vi "MB_TCP_NS300.vi"(5 "Status Reference":T1, 6 "N":i32, 7 "Data Reference":T2, 9 "timeouts":T3={"conn_timeout"=1000, "reconn_timeout"=3000, "N attempt max"=3, "t_reset_TTL"=120000, "write_timeout"=10, "read_timeout"=500, "period"=100} {"t_reset_TTL" min=10 max=240000 step=1; "period" min=10 max=100000 step=1; "read_timeout" min=10 max=60000 step=1; "write_timeout" min=1 max=60000 step=1; "N attempt max" min=1 max=5 step=1; "reconn_timeout" min=10 max=240000 step=1; "conn_timeout" min=10 max=240000}, 10 "write enable":bool=TRUE, 11 "stop":bool) -> (0 "error out":errorcluster, 2 "errors":i32, 3 "Z3":u32)   [LabVIEW 2019, in "MB_TCP1.lvlib"]
uses:
  MB_TCP1.lvlib
  Timer Delay/Timers.lvlib
  NI_modbus_upd/NI_modbus_upd.lvlib
  NI_modbus_upd/MB Modbus Command.ctl
  ICPCON Registers/ICPCON Registers.lvlib
  ICPCON Status/ICPCON Status.lvlib
  Timer Delay/unix time 1ms.vi
  NI_modbus_upd/TCP/TCP.lvclass
  ICPCON Registers/Ctl/ICPCON Data.ctl
  ICPCON Status/Ctl/ICPCON Status.ctl
panel:
  out "stopped":bool
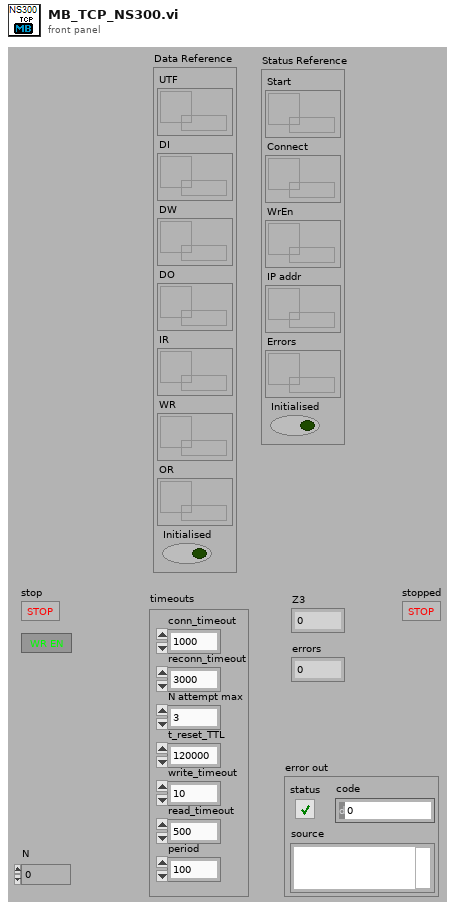
[diagram p1: front panel]
types:
  T1 = typedef "ICPCON Status.lvlib/ICPCON Status.ctl" = cluster{"Start":refnum<data-value>, "Connect":refnum<data-value>, "WrEn":refnum<data-value>, "IP addr":refnum<data-value>, "Errors":refnum<data-value>, "Initialised":bool}
  T2 = typedef "ICPCON Registers.lvlib/ICPCON Data.ctl" = cluster{"UTF":refnum<data-value>, "DI":refnum<data-value>, "DW":refnum<data-value>, "DO":refnum<data-value>, "IR":refnum<data-value>, "WR":refnum<data-value>, "OR":refnum<data-value>, "Initialised":bool}
  T3 = cluster{"conn_timeout":i32, "reconn_timeout":i32, "N attempt max":i32, "t_reset_TTL":i32, "write_timeout":i32, "read_timeout":i32, "period":i32}
  T4 = typedef "NI_modbus_upd.lvlib/MB Modbus Command.ctl" = cluster{"Function Code":u8, "Starting Address":u16, "Quantity":u16, "Data":u16[], "Discrete":bool[]}
  T5 = cluster{"Transaction ID":u16, "Protocol ID":u16, "Length":u16, "Unit ID":u8}
  T6 = cluster{"Remote IP Address":string, "Remote Port":u16}
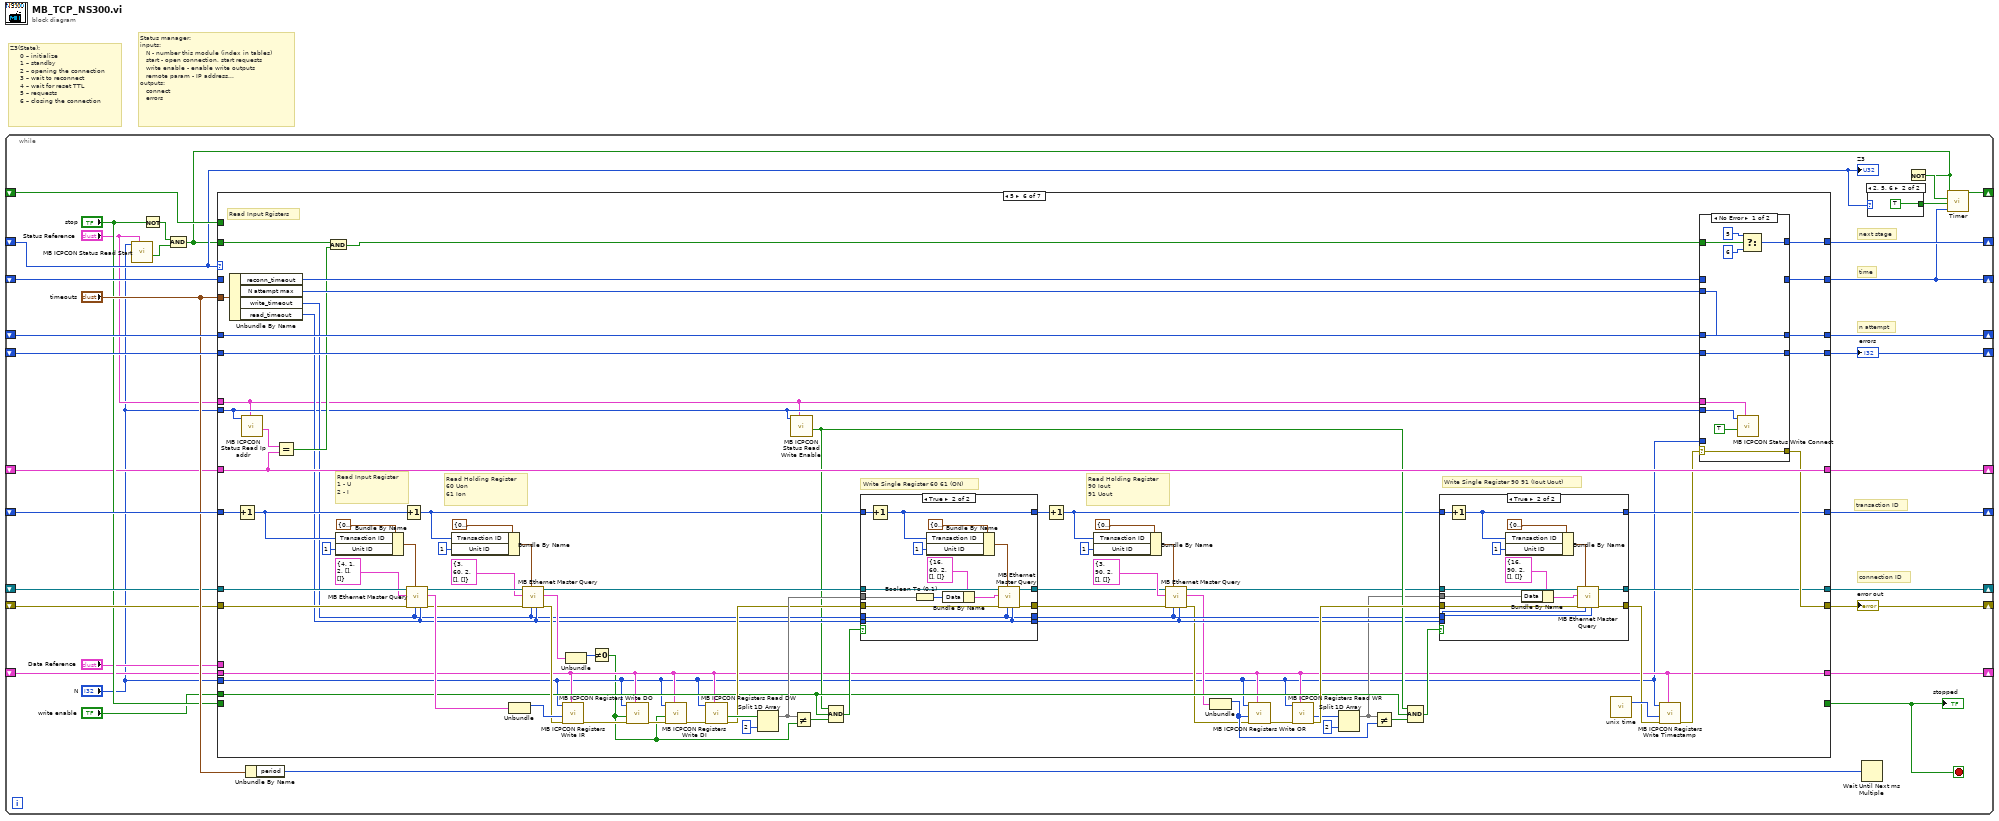
[diagram p0: block diagram]
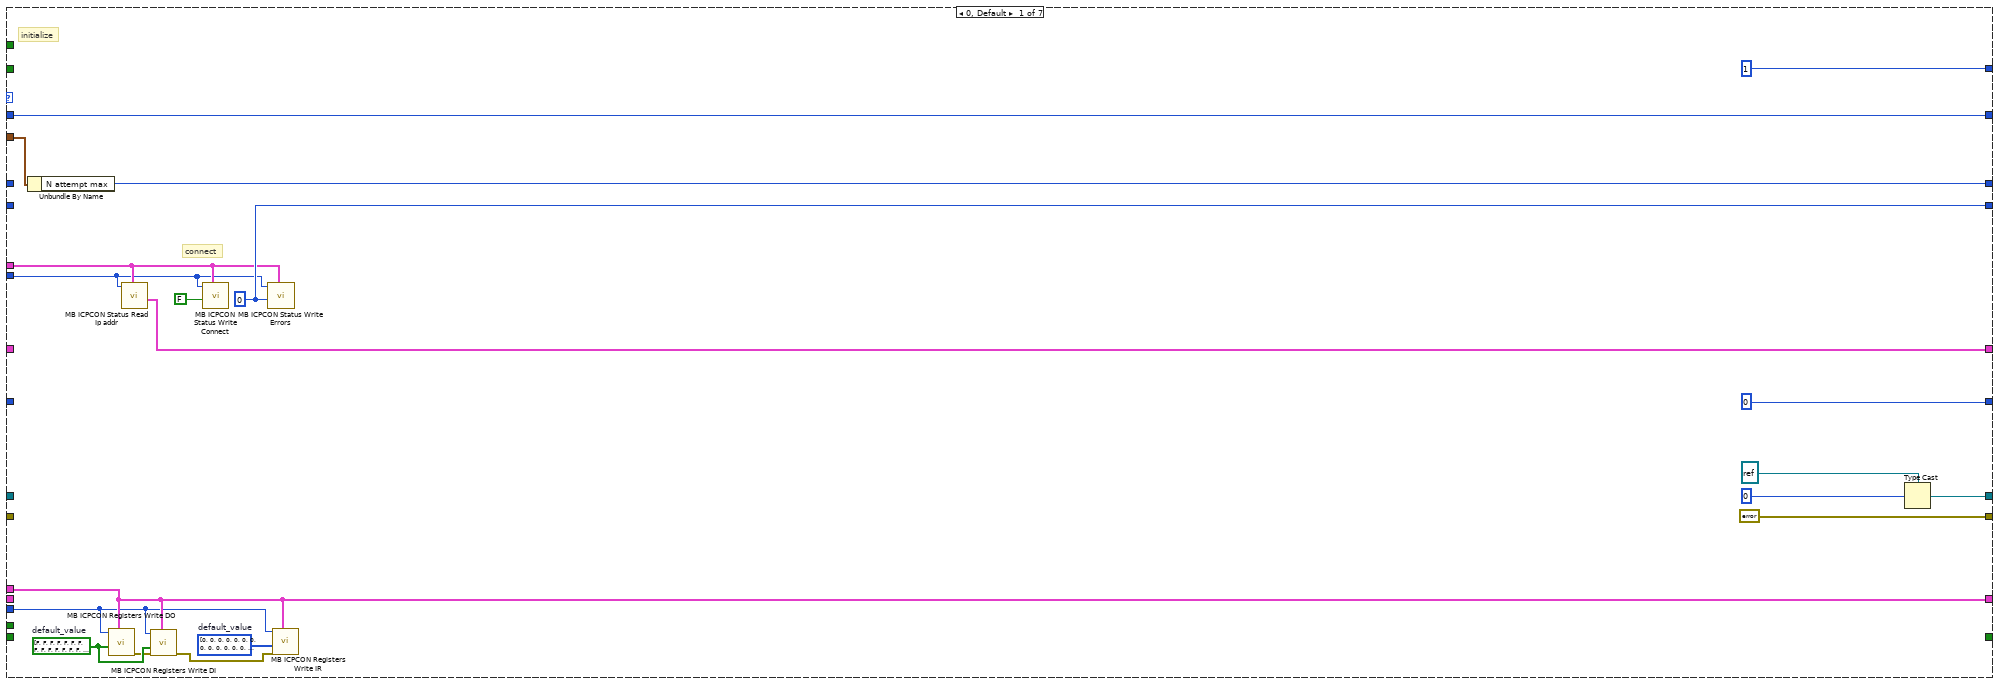
[diagram p2: hidden frame]
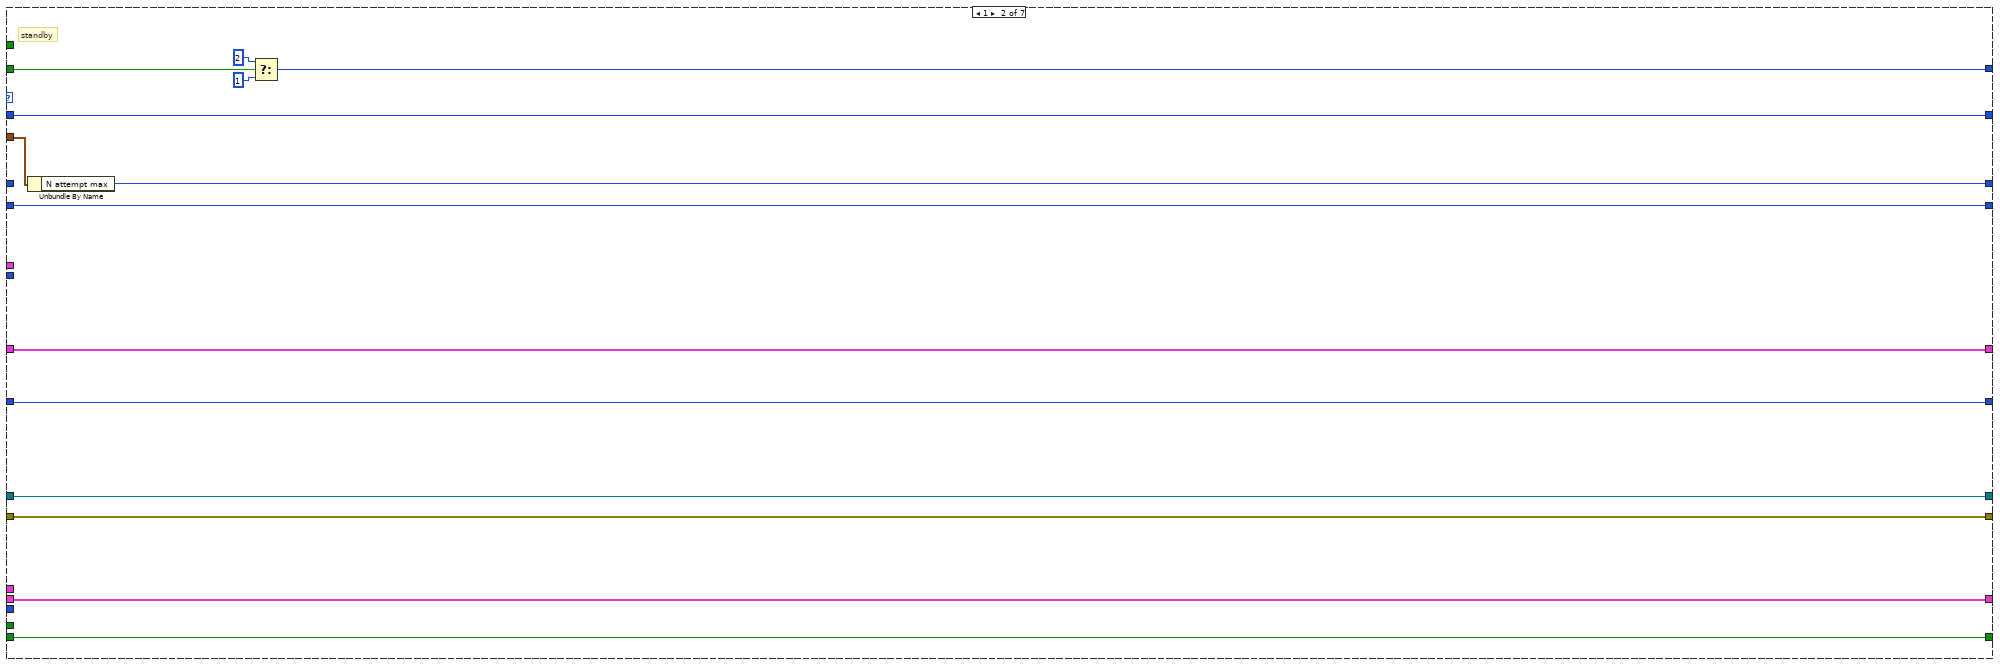
[diagram p3: hidden frame]
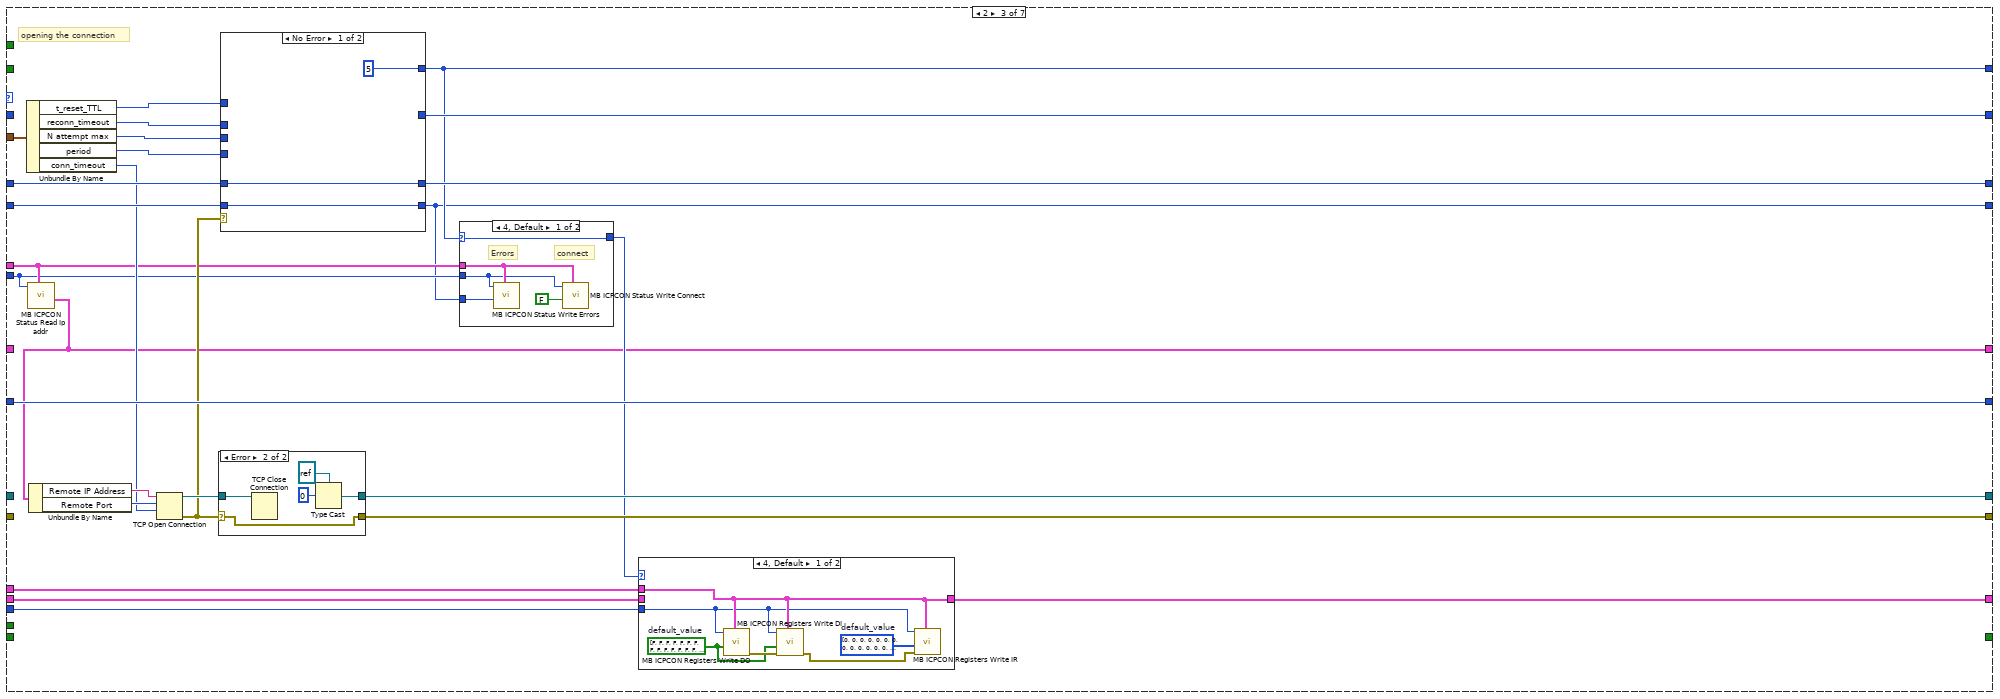
[diagram p4: hidden frame]
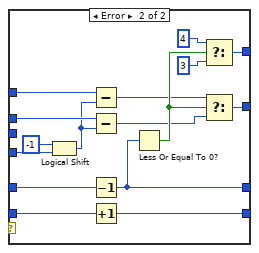
[diagram p8: hidden frame]
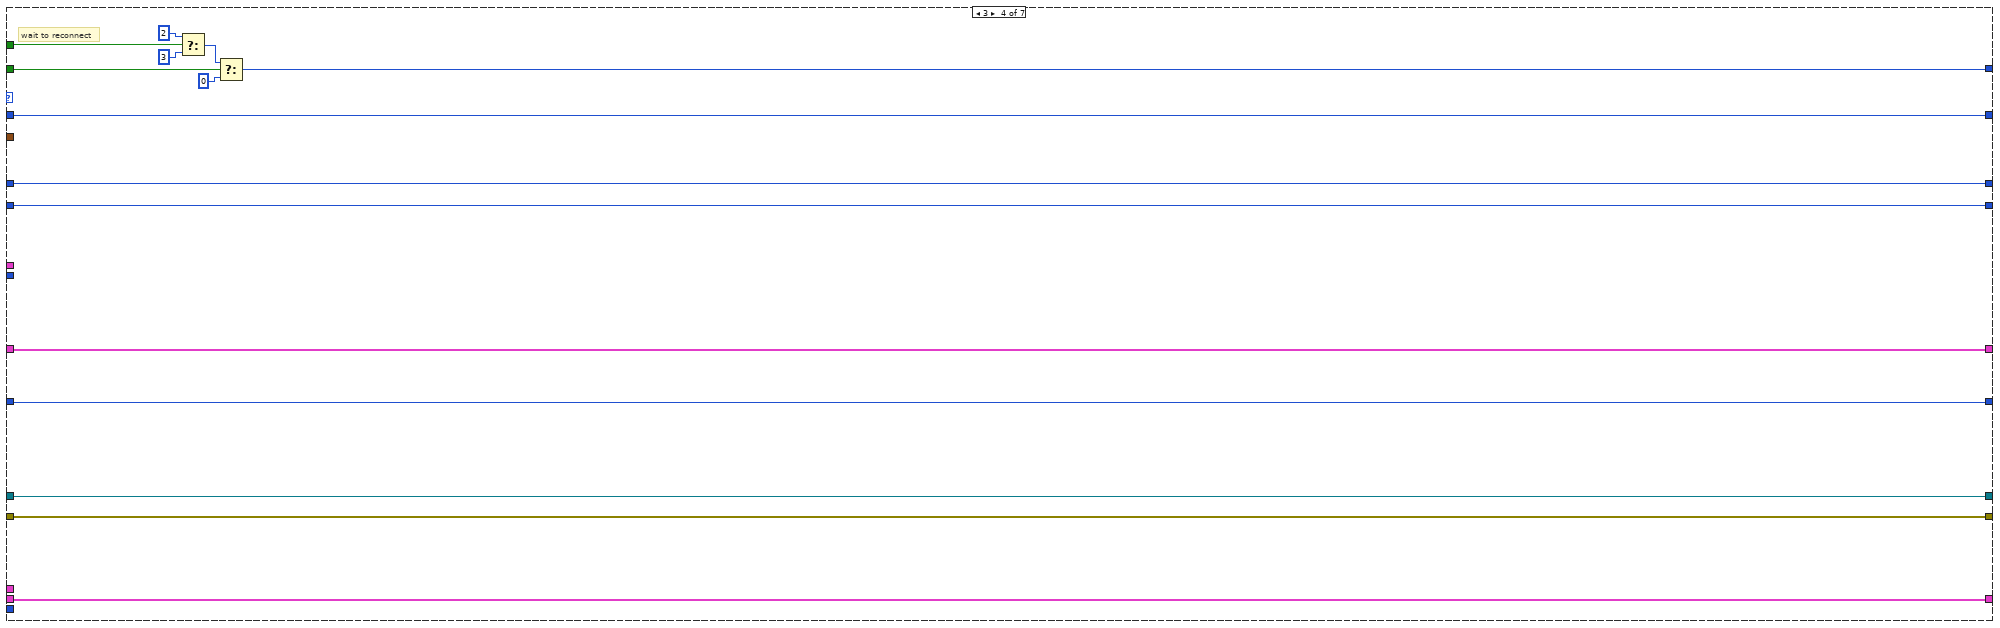
[diagram p9: hidden frame]
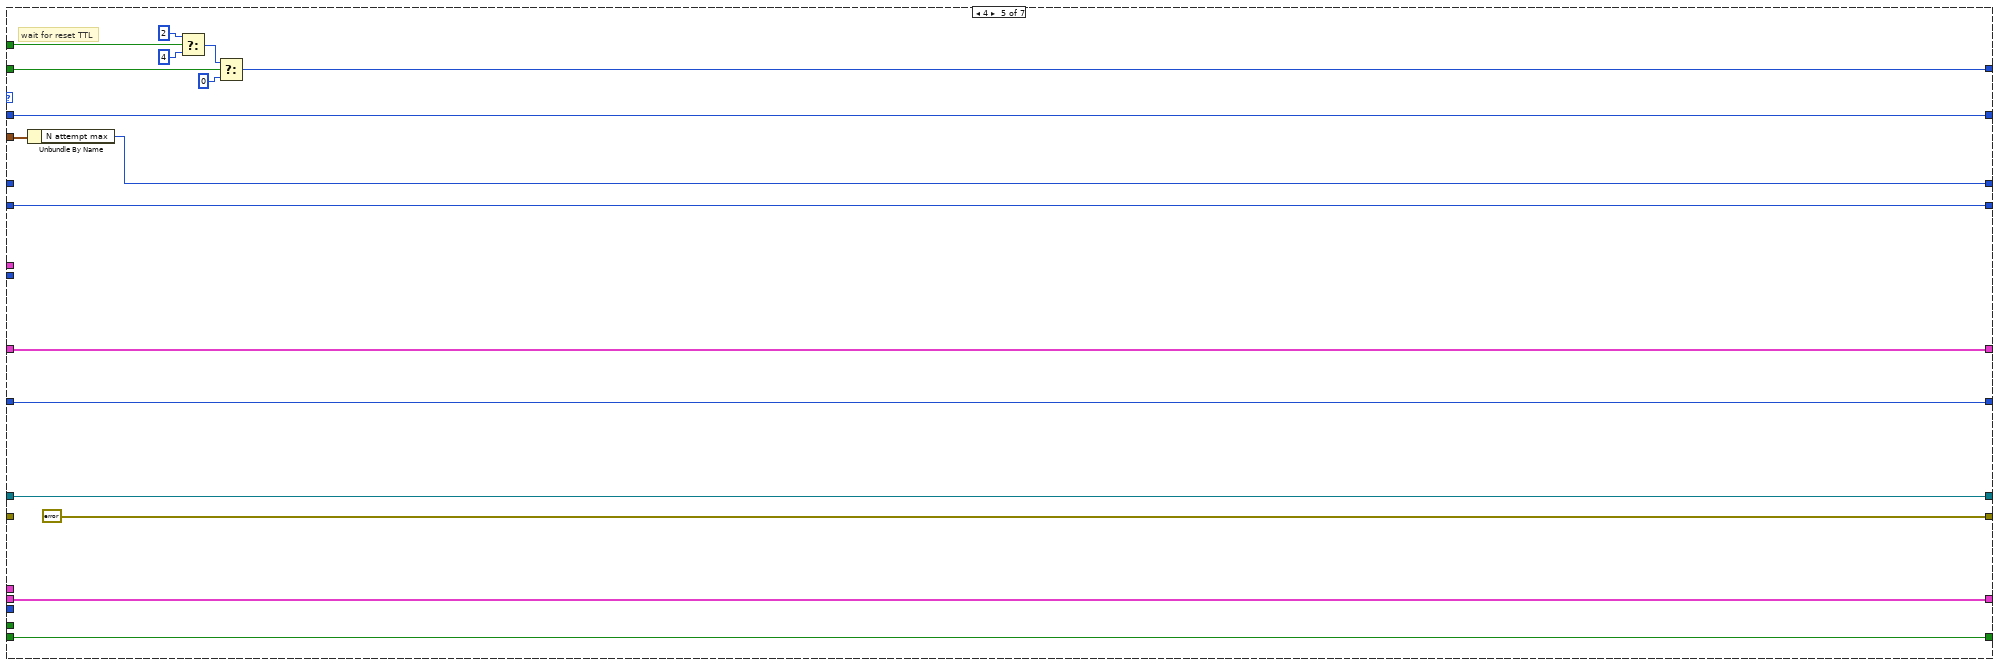
[diagram p10: hidden frame]
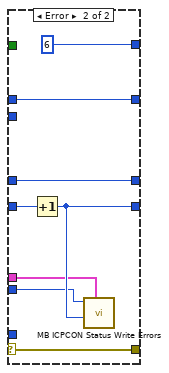
[diagram p13: hidden frame]
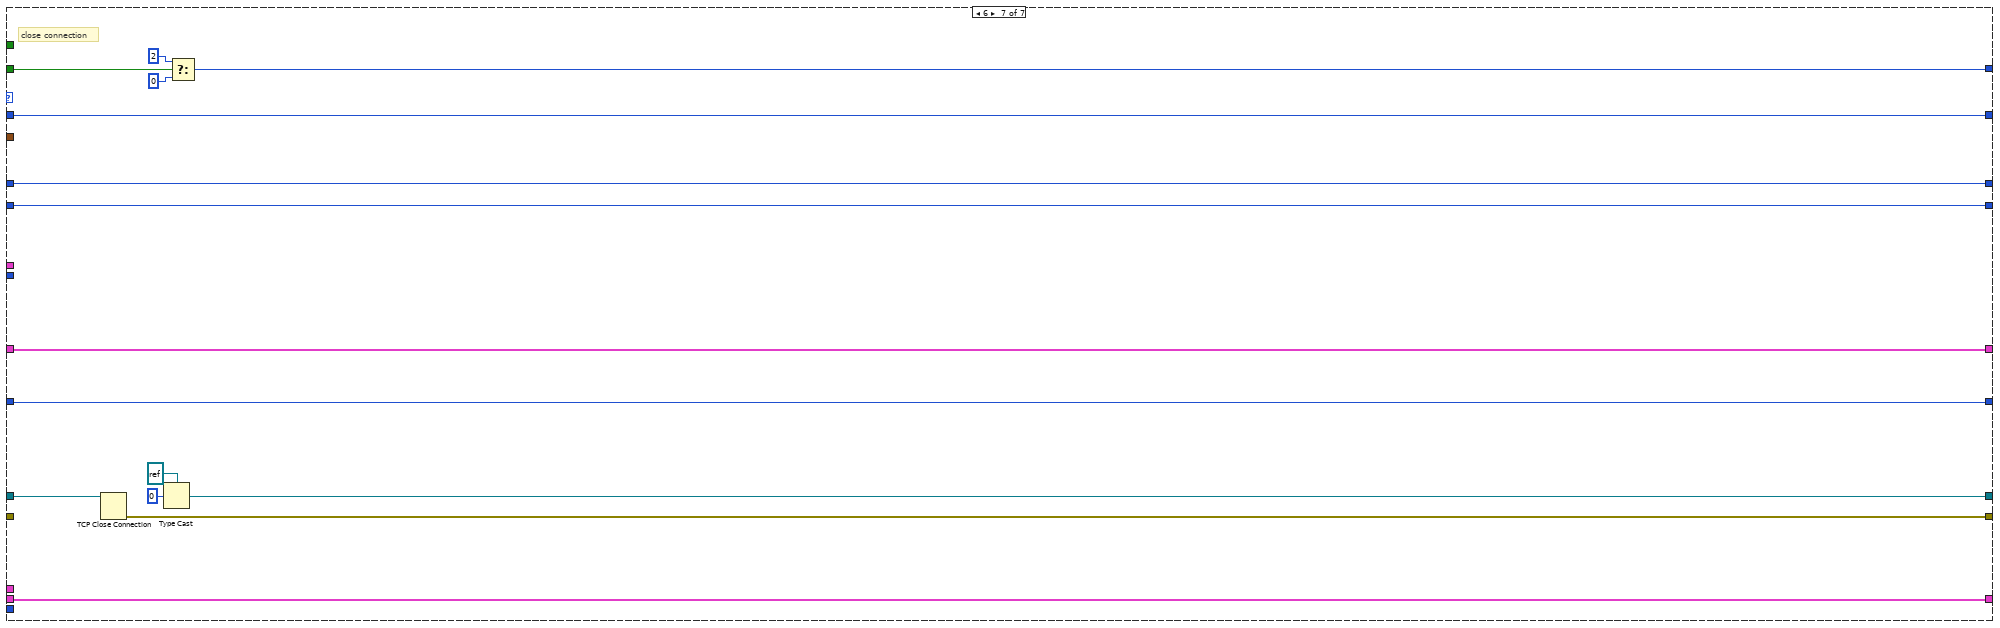
[diagram p14: hidden frame]
diagram:
  # "Status manager:\ninputs:\n   N - number this module (index in tables)\n   start - open connection, start requests\n   write enable - enable write outputs\n   remote param - IP address...\noutputs:\n   connect\n   errors"
  # "Z3(State):\n     0 – initialize \n     1 – standby\n     2 – opening the connection\n     3 – wait to reconnect\n     4 – wait for reset TTL\n     5 – requests\n     6 – closing the connection"
  n1 = while {
    shift-right: [w18] -> _
    shift-left: _ -> [w14]
    shift-right: [w17] -> _
    shift-left: _ -> [w32]
    shift-right: [w31] -> _
    shift-left: _ -> [w29]
    shift-right: [w30] -> _
    shift-left: _ -> [w28]
    shift-right: [w27] -> _
    shift-left: _ -> [w19]
    shift-right: [w26] -> _
    shift-left: _ -> [w20]
    shift-right: [w25] -> _
    shift-left: _ -> [w24]
    shift-right: [w16] -> _
    shift-left: _ -> [w15]
    shift-right: [w10] -> _
    shift-left: _ -> [w9]
    shift-right: [w7] -> _
    shift-left: _ -> [w6]
    stop <- w1 stop-if-true
    # "connection ID"
    # "transaction ID"
    # "n attempt"
    # "time"
    # "next stage"
    n2 = call "MB ICPCON Status Read Start.vi"("Status Reference"="Status Reference", "N"="N") -> ("Start"=w4:bool)  [unwired: 8 in, 1 out]
    n3 = Not(x="stop") -> (.not. x?=w12:bool)
    n4 = And(x=w12, y=w4) -> (x .and. y?=w13:bool)
    n5 = case shown="5" w14 {
      tunnel: [w51 w59 w80 w146 w151 w195 w312] -> w27
      tunnel: [errorcluster {"status"=FALSE, "code"=0, "source"=""} ("error out") w58 w78 w145 errorcluster {"status"=FALSE, "code"=0, "source"=""} ("error out") w215 w313] -> w26
      tunnel: w19 -> [_ w59 _ w146 w151 w235 w309]
      tunnel: w20 -> [_ w58 _ w145 _ w234 _]
      tunnel: w24 -> [_ w67 w94 w148 w165 w244 w314]
      tunnel: [u16 0 ("x") w67 w94 w148 w165 w196 w314] -> w25
      tunnel: [w46 w63 w90 w147 w161 w242 w306] -> w31
      tunnel: w29 -> [_ _ w91 w147 _ w242 w306]
      tunnel: [w41 w66 w68 w144 w164 w241 w311] -> w30
      tunnel: w28 -> [_ w66 w93 w144 w164 w240 w311]
      tunnel: [w48 w65 w87 w143 w163 w237 w310] -> w17
      tunnel: w32 -> [w48 w65 _ w143 w163 _ w310]
      tunnel: "timeouts" -> [w47 w64 w92 _ w162 w243 _]
      tunnel: w13 -> [_ w57 _ w139 w153 w229 w307]
      tunnel: [u32 1 w60 w77 w136 w156 w236 w302] -> w18
      tunnel: w15 -> [_ _ _ w137 w155 _ _]
      tunnel: "N" -> [w37 _ w74 _ _ w167 _]
      tunnel: "stop" -> [_ w56 _ _ w152 _ _]
      tunnel: [_ w56 _ _ w152 _ _] -> w1
      tunnel: [w42 w55 w71 w135 w150 w227 w301] -> w10
      tunnel: w9 -> [_ w55 _ w135 w150 w227 w301]
      tunnel: "Data Reference" -> [w38 _ w73 _ _ _ _]
      tunnel: [w38 w54 w76 w134 w149 w168 w300] -> w7
      tunnel: w6 -> [_ w54 w72 w134 w149 w168 w300]
      tunnel: "write enable" -> [_ _ _ _ _ w192 _]
      tunnel: "Status Reference" -> [w40 _ w70 _ _ w201 _]
      tunnel: "N" -> [w39 _ w69 _ _ w202 _]
      frame 0, Default {
        w41 = 0 ("N attempt max")
        w36 = bool[] [FALSE, FALSE, FALSE, FALSE, FALSE, FALSE, FALSE, FALSE, FALSE, FALSE, FALSE, FALSE, FALSE, FALSE, FALSE, FALSE, FALSE, FALSE, FALSE, FALSE, FALSE, FALSE, FALSE, FALSE, FALSE, FALSE, FALSE, FALSE, FALSE, FALSE, FALSE, FALSE]  # default_value
        w44 = u16[] [0, 0, 0, 0, 0, 0, 0, 0, 0, 0, 0, 0, 0, 0, 0, 0, 0, 0, 0, 0]  # default_value
        # "connect"
        # "initialize"
        n6 = Unbundle By Name(w47) -> ("N attempt max"=w46:i32)
        n7 = call "MB ICPCON Registers Write DO.vi"("Data Reference"=w38, "Bits In"=w36, "N"=w37) -> ("error out"=w35:errorcluster)  [unwired: 8 in]
        n8 = call "MB ICPCON Status Read Ip addr.vi"("Status Reference"=w40, "N"=w39) -> ("IP address"=w42:T6)  [unwired: 8 in, 1 out]
        n9 = call "MB ICPCON Registers Write DI.vi"("Data Reference"=w38, "error in (no error)"=w35, "Bits In"=w36, "N"=w37) -> ("error out"=w34:errorcluster)  [unwired: 7 in]
        n10 = call "MB ICPCON Status Write Connect.vi"("Status Reference"=w40, "Connect"=FALSE ("connect"), "N"=w39) -> ()  [unwired: 8 in, 1 out]
        n11 = call "MB ICPCON Status Write Errors.vi"("Status Reference"=w40, "Errors"=w41, "N"=w39) -> ()  [unwired: 8 in, 1 out]
        n12 = call "MB ICPCON Registers Write IR.vi"("Data Reference"=w38, "error in (no error)"=w34, "Words In"=w44, "N"=w37) -> ()  [unwired: 7 in, 1 out]
        n13 = Type Cast(type=refnum<k5> refnum ("connection ID"), x=u32 0) -> (*(type *) &x=w51:refnum<k5>)
      }
      frame 1 {
        # "standby"
        n14 = Unbundle By Name(w64) -> ("N attempt max"=w63:i32)
        n15 = Select(t=u32 2, s=w57, f=u32 1) -> (s? t:f=w60:u32)
      }
      frame 2 {
        # "opening the connection"
        n16 = Unbundle By Name(w92) -> ("t_reset_TTL"=w86:i32, "reconn_timeout"=w88:i32, "N attempt max"=w89:i32, "period"=w83:i32, "conn_timeout"=w82:i32)
        n17 = call "MB ICPCON Status Read Ip addr.vi"("Status Reference"=w70, "N"=w69) -> ("IP address"=w71:T6)  [unwired: 8 in, 1 out]
        n18 = Unbundle By Name(w71) -> ("Remote IP Address"=w85:string, "Remote Port"=w84:u16)
        n19 = TCP Open Connection(address=w85, remote port or service name=w84, timeout ms (60000)=w82) -> (connection ID=w81:refnum<k5>, error out=w79:errorcluster)  [unwired: 2 in]
        n20 = case shown="Error" w79 {
          selector: w79 -> [w108 w110]
          tunnel: w81 -> [w109 w113]
          tunnel: [w109 w112] -> w80
          tunnel: [w108 w110] -> w78
          frame No Error {
          }
          frame Error {
            n21 = TCP Close Connection(connection ID=w113) -> ()  [unwired: 2 in, 2 out]
            n22 = Type Cast(type=refnum<k5> refnum ("connection ID"), x=u32 0) -> (*(type *) &x=w112:refnum<k5>)
          }
        }
        n23 = case shown="No Error" w79 {
          tunnel: w93 -> [w117 w133]
          tunnel: [w117 w132] -> w68
          tunnel: w91 -> [w116 w131]
          tunnel: [w116 w130] -> w90
          tunnel: w89 -> [_ _]
          tunnel: [u32 5 w127] -> w77
          tunnel: w88 -> [_ w126]
          tunnel: [_ w125] -> w87
          tunnel: w86 -> [_ w122]
          tunnel: w83 -> [_ w120]
          frame No Error {
          }
          frame Error {
            n24 = Logical Shift(y=i16 -1, x=w120) -> (x << y=w118:i32)
            n25 = Subtract(x=w122, y=w118) -> (x-y=w121:i32)
            n26 = Subtract(x=w126, y=w118) -> (x-y=w123:i32)
            n27 = Decrement(x=w131) -> (x-1=w130:i32)
            n28 = Increment(x=w133) -> (x+1=w132:i32)
            n29 = Less Or Equal To 0?(x=w130) -> (x <= 0?=w124:bool)
            n30 = Select(t=u32 4, s=w124, f=u32 3) -> (s? t:f=w127:u32)
            n31 = Select(t=w121, s=w124, f=w123) -> (s? t:f=w125:i32)
          }
        }
        n32 = case shown="4, Default" w77 {
          selector: w77 -> [w106 w107]
          tunnel: [w106 w107] -> w75
          tunnel: w70 -> [w104 _]
          tunnel: w69 -> [w103 _]
          tunnel: w68 -> [w102 _]
          frame 4, Default {
            # "Errors"
            # "connect"
            n33 = call "MB ICPCON Status Write Errors.vi"("Status Reference"=w104, "Errors"=w102, "N"=w103) -> ()  [unwired: 8 in, 1 out]
            n34 = call "MB ICPCON Status Write Connect.vi"("Status Reference"=w104, "Connect"=FALSE ("f"), "N"=w103) -> ()  [unwired: 8 in, 1 out]
          }
          frame 3, 5 {
          }
        }
        n35 = case shown="4, Default" w75 {
          tunnel: w74 -> [w98 _]
          tunnel: w72 -> [_ w101]
          tunnel: [w99 w101] -> w76
          tunnel: w73 -> [w99 _]
          frame 4, Default {
            w95 = bool[] [FALSE, FALSE, FALSE, FALSE, FALSE, FALSE, FALSE, FALSE, FALSE, FALSE, FALSE, FALSE, FALSE, FALSE, FALSE, FALSE, FALSE, FALSE, FALSE, FALSE, FALSE, FALSE, FALSE, FALSE, FALSE, FALSE, FALSE, FALSE, FALSE, FALSE, FALSE, FALSE]  # default_value
            w100 = u16[] [0, 0, 0, 0, 0, 0, 0, 0, 0, 0, 0, 0, 0, 0, 0, 0, 0, 0, 0, 0]  # default_value
            n36 = call "MB ICPCON Registers Write DO.vi"("Data Reference"=w99, "Bits In"=w95, "N"=w98) -> ("error out"=w97:errorcluster)  [unwired: 8 in]
            n37 = call "MB ICPCON Registers Write DI.vi"("Data Reference"=w99, "error in (no error)"=w97, "Bits In"=w95, "N"=w98) -> ("error out"=w96:errorcluster)  [unwired: 7 in]
            n38 = call "MB ICPCON Registers Write IR.vi"("Data Reference"=w99, "error in (no error)"=w96, "Words In"=w100, "N"=w98) -> ()  [unwired: 7 in, 1 out]
          }
          frame 3, 5 {
          }
        }
      }
      frame 3 {
        # "wait to reconnect"
        n39 = Select(t=u32 2, s=w137, f=u32 3) -> (s? t:f=w138:u32)
        n40 = Select(t=w138, s=w139, f=u32 0) -> (s? t:f=w136:u32)
      }
      frame 4 {
        # "wait for reset TTL"
        n41 = Unbundle By Name(w162) -> ("N attempt max"=w161:i32)
        n42 = Select(t=u32 2, s=w155, f=u32 4) -> (s? t:f=w157:u32)
        n43 = Select(t=w157, s=w153, f=u32 0) -> (s? t:f=w156:u32)
      }
      frame 5 {
        # "Read Holding Register\n90 Iout\n91 Uout"
        # "Write Single Register 60 61 (ON)"
        # "Write Single Register 90 91 (Iout Uout)"
        # "Read Holding Register\n60 Uon\n61 Ion"
        # "Read Input Register\n1 - U\n2 - I"
        # "Read Input Rgisters"
        n44 = Unbundle By Name(w243) -> ("reconn_timeout"=w238:i32, "N attempt max"=w239:i32, "write_timeout"=w205:i32, "read_timeout"=w206:i32)
        n45 = Increment(x=w244) -> (x+1=w222:u16)
        n46 = call "MB ICPCON Status Read Ip addr.vi"("Status Reference"=w201, "N"=w202) -> ("IP address"=w213:T6)  [unwired: 8 in, 1 out]
        n47 = Equal?(x=w213, y=w227) -> (x = y?=w226:bool)
        n48 = And(x=w229, y=w226) -> (x .and. y?=w228:bool)
        n49 = Bundle By Name(cluster=T5 {"Transaction ID"=0, "Protocol ID"=0, "Length"=0, "Unit ID"=0} ("MBAP Header"), "Transaction ID"=w222, "Unit ID"=u8 1) -> (w230:T5)
        n50 = Increment(x=w222) -> (x+1=w204:u16)
        n51 = call "MB Ethernet Master Query.vi"(4:w206, 6:w205, "MBAP Header"=w230, "error in (no error)"=w234, "Modbus Command"=T4 {"Function Code"=4, "Starting Address"=1, "Quantity"=2, "Data"=[], "Discrete"=[]} ("MODBUS Command"), "TCP in"=w235) -> ("error out"=w221:errorcluster, "Registers"=w233:cluster{"Registers":u16[], "Discrete":bool[]}, "TCP out"=w219:refnum<class "TCP.lvclass">)  [unwired: 2 in, 1 out]
        n52 = Bundle By Name(cluster=T5 {"Transaction ID"=0, "Protocol ID"=0, "Length"=0, "Unit ID"=0} ("MBAP Header"), "Transaction ID"=w204, "Unit ID"=u8 1) -> (w225:T5)
        n53 = Unbundle(w233) -> ("Registers"=w217:u16[])  [unwired: 1 out]
        n54 = call "MB Ethernet Master Query.vi"(4:w206, 6:w205, "MBAP Header"=w225, "error in (no error)"=w221, "Modbus Command"=T4 {"Function Code"=3, "Starting Address"=60, "Quantity"=2, "Data"=[], "Discrete"=[]} ("MODBUS Command"), "TCP in"=w219) -> ("error out"=w216:errorcluster, "Registers"=w220:cluster{"Registers":u16[], "Discrete":bool[]}, "TCP out"=w203:refnum<class "TCP.lvclass">)  [unwired: 2 in, 1 out]
        n55 = call "MB ICPCON Registers Write IR.vi"("Data Reference"=w168, "error in (no error)"=w216, "Words In"=w217, "N"=w167) -> ("error out"=w218:errorcluster)  [unwired: 7 in]
        n56 = Unbundle(w220) -> ("Registers"=w197:u16[])  [unwired: 1 out]
        n57 = Not Equal To 0?(x=w197) -> (x != 0?=w166:bool[])
        n58 = call "MB ICPCON Registers Write DO.vi"("Data Reference"=w168, "error in (no error)"=w218, "Bits In"=w166, "N"=w167) -> ("error out"=w170:errorcluster)  [unwired: 7 in]
        n59 = call "MB ICPCON Registers Write DI.vi"("Data Reference"=w168, "error in (no error)"=w170, "Bits In"=w166, "N"=w167) -> ("error out"=w169:errorcluster)  [unwired: 7 in]
        n60 = call "MB ICPCON Registers Read DW.vi"("Data Reference"=w168, "error in (no error)"=w169, "N"=w167) -> ("error out"=w207:errorcluster, "Bits out"=w210:bool[])  [unwired: 7 in]
        n61 = Split 1D Array(array=w210, index=2 ("length")) -> (first subarray=w208:bool[])  [unwired: 1 out]
        n62 = call "MB ICPCON Status Read Write Enable.vi"("Status Reference"=w201, "N"=w202) -> ("Write Enable"=w190:bool)  [unwired: 8 in, 1 out]
        n63 = Not Equal?(x=w208, y=w166) -> (x != y?=w212:bool)
        n64 = Compound Arithmetic op=AND(w190, w192, w212) -> (w211:bool)
        n65 = case shown="True" w211 {
          tunnel: w206 -> [w246 w252]
          tunnel: w205 -> [w245 w251]
          tunnel: w204 -> [w248 w262]
          tunnel: [w248 w253] -> w185
          tunnel: w207 -> [w247 w260]
          tunnel: [w247 w254] -> w175
          tunnel: w203 -> [w249 w259]
          tunnel: [w249 w255] -> w183
          tunnel: w208 -> [_ w250]
          tunnel: [w246 w252] -> w180
          tunnel: [w245 w251] -> w181
          frame False {
          }
          frame True {
            n66 = Increment(x=w262) -> (x+1=w253:u16)
            n67 = Boolean To (0,1)(Boolean=w250) -> (0, 1=w256:i16[])
            n68 = Bundle By Name(cluster=T5 {"Transaction ID"=0, "Protocol ID"=0, "Length"=0, "Unit ID"=0} ("MBAP Header"), "Transaction ID"=w253, "Unit ID"=u8 1) -> (w263:T5)
            n69 = Bundle By Name(cluster=T4 {"Function Code"=16, "Starting Address"=60, "Quantity"=2, "Data"=[], "Discrete"=[]} ("MODBUS Command"), "Data"=w256) -> (w258:T4)
            n70 = call "MB Ethernet Master Query.vi"(4:w252, 6:w251, "MBAP Header"=w263, "error in (no error)"=w260, "Modbus Command"=w258, "TCP in"=w259) -> ("error out"=w254:errorcluster, "TCP out"=w255:refnum<class "TCP.lvclass">)  [unwired: 2 in, 2 out]
          }
        }
        n71 = Increment(x=w185) -> (x+1=w184:u16)
        n72 = Bundle By Name(cluster=T5 {"Transaction ID"=0, "Protocol ID"=0, "Length"=0, "Unit ID"=0} ("MBAP Header"), "Transaction ID"=w184, "Unit ID"=u8 1) -> (w186:T5)
        n73 = call "MB Ethernet Master Query.vi"(4:w180, 6:w181, "MBAP Header"=w186, "error in (no error)"=w175, "Modbus Command"=T4 {"Function Code"=3, "Starting Address"=90, "Quantity"=2, "Data"=[], "Discrete"=[]} ("MODBUS Command"), "TCP in"=w183) -> ("error out"=w172:errorcluster, "Registers"=w177:cluster{"Registers":u16[], "Discrete":bool[]}, "TCP out"=w182:refnum<class "TCP.lvclass">)  [unwired: 2 in, 1 out]
        n74 = Unbundle(w177) -> ("Registers"=w174:u16[])  [unwired: 1 out]
        n75 = call "MB ICPCON Registers Write OR.vi"("Data Reference"=w168, "error in (no error)"=w172, "Words In"=w174, "N"=w167) -> ("error out"=w173:errorcluster)  [unwired: 7 in]
        n76 = call "MB ICPCON Registers Read WR.vi"("Data Reference"=w168, "error in (no error)"=w173, "N"=w167) -> ("error out"=w193:errorcluster, "Words out"=w178:u16[])  [unwired: 7 in]
        n77 = Split 1D Array(array=w178, index=2 ("length")) -> (first subarray=w176:u16[])  [unwired: 1 out]
        n78 = Not Equal?(x=w176, y=w174) -> (x != y?=w171:bool)
        n79 = Compound Arithmetic op=AND(w190, w192, w171) -> (w191:bool)
        n80 = case shown="True" w191 {
          tunnel: w180 -> [_ w274]
          tunnel: w181 -> [_ w273]
          tunnel: w184 -> [w266 w279]
          tunnel: [w266 w269] -> w196
          tunnel: w193 -> [w265 w277]
          tunnel: [w265 w268] -> w194
          tunnel: w182 -> [w267 w276]
          tunnel: [w267 w270] -> w195
          tunnel: w176 -> [_ w271]
          frame False {
          }
          frame True {
            n81 = Increment(x=w279) -> (x+1=w269:u16)
            n82 = Bundle By Name(cluster=T5 {"Transaction ID"=0, "Protocol ID"=0, "Length"=0, "Unit ID"=0} ("MBAP Header"), "Transaction ID"=w269, "Unit ID"=u8 1) -> (w280:T5)
            n83 = Bundle By Name(cluster=T4 {"Function Code"=16, "Starting Address"=90, "Quantity"=2, "Data"=[], "Discrete"=[]} ("MODBUS Command"), "Data"=w271) -> (w275:T4)
            n84 = call "MB Ethernet Master Query.vi"(4:w274, 6:w273, "MBAP Header"=w280, "error in (no error)"=w277, "Modbus Command"=w275, "TCP in"=w276) -> ("error out"=w268:errorcluster, "TCP out"=w270:refnum<class "TCP.lvclass">)  [unwired: 2 in, 2 out]
          }
        }
        n85 = call-poly "unix time.vi"() -> ("unix time (ms)"=w214:u64)  [unwired: 2 in, 1 out]
        n86 = call "MB ICPCON Registers Write Timestamp.vi"("Data Reference"=w168, "error in (no error)"=w194, "UTF"=w214, "N"=w167) -> ("error out"=w200:errorcluster)  [unwired: 7 in]
        n87 = case shown="No Error" w200 {
          selector: w200 -> [w285 w295]
          tunnel: w240 -> [w286 w299]
          tunnel: [w286 w294] -> w241
          tunnel: [w288 u32 6] -> w236
          tunnel: w242 -> [_ w297]
          tunnel: w239 -> [w291 _]
          tunnel: [w291 w297] -> _
          tunnel: w238 -> [_ w296]
          tunnel: [_ w296] -> w237
          tunnel: w228 -> [w287 _]
          tunnel: w167 -> [_ _]
          tunnel: [w285 w295] -> w215
          tunnel: w201 -> [w283 w293]
          tunnel: w202 -> [w282 w292]
          frame No Error {
            n88 = call "MB ICPCON Status Write Connect.vi"("Status Reference"=w283, "Connect"=TRUE ("f"), "N"=w282) -> ()  [unwired: 8 in, 1 out]
            n89 = Select(t=u32 5, s=w287, f=u32 6) -> (s? t:f=w288:u32)
          }
          frame Error {
            n90 = Increment(x=w299) -> (x+1=w294:i32)
            n91 = call "MB ICPCON Status Write Errors.vi"("Status Reference"=w293, "Errors"=w294, "N"=w292) -> ()  [unwired: 8 in, 1 out]
          }
        }
      }
      frame 6 {
        # "close connection"
        n92 = TCP Close Connection(connection ID=w309) -> (error out=w313:errorcluster)  [unwired: 2 in, 1 out]
        n93 = Type Cast(type=refnum<k5> refnum ("connection ID"), x=u32 0) -> (*(type *) &x=w312:refnum<k5>)
        n94 = Select(t=u32 2, s=w307, f=u32 0) -> (s? t:f=w302:u32)
      }
    }
    "error out" <- w26
    "errors" <- w30
    "stopped" <- w1
    n95 = Unbundle By Name("timeouts") -> ("period"=w22:i32)
    n96 = Wait Until Next ms Multiple(millisecond multiple=w22) -> ()  [unwired: 1 out]
    n97 = case shown="2, 5, 6" w14 {
      tunnel: [_ TRUE] -> w21
      frame 0, Default {
      }
      frame 2, 5, 6 {
      }
    }
    n98 = Not(x=w13) -> (.not. x?=w33:bool)
    n99 = call "Timer.vi"("ms"=w17, "Load (F)"=w21, "Reset (F)"=w33, "Start (T)"=w13) -> ("End"=w16:bool)  [unwired: 5 in, 1 out]
    "Z3" <- w14
  }
